vi "GetAllPositions.vi"(8 "error In":errorcluster, 9 "Device Address In":i32, 10 "DeviceKey In":string, 11 "CmdLib In":refnum<k24>) -> (0 "error out":errorcluster, 1 "Device Address Out":i32, 2 "DeviceKey Out":string, 3 "CmdLib Out":refnum<k24>, 4 "Positions":i32[](array[numeric]))   [LabVIEW 2013]
uses:
  C:/GEECS/Developers Version/source/Device Driver/Picomotor8742dotNet/NewFocus/CmdLib.dll
  CmdLib.dll
panel:
  # "Position Motor 1"
  # "Position Motor 2"
  # "Position Motor 3"
  # "Position Motor 4"
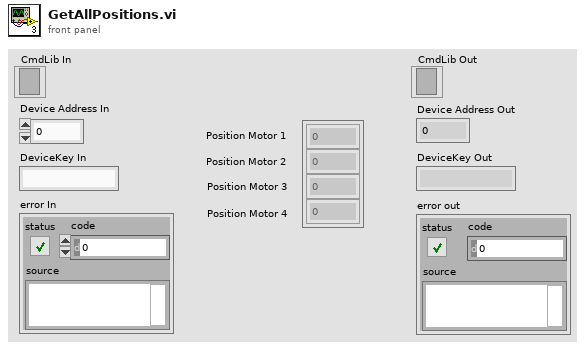
[diagram p1: front panel]
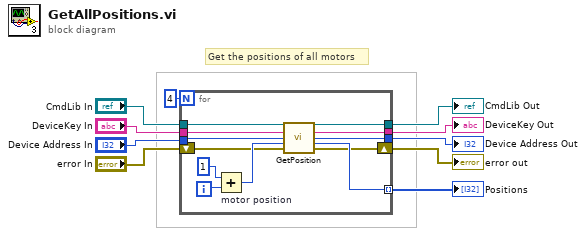
[diagram p0: block diagram]
diagram:
  # "Get the positions of all motors"
  n1 = for {
    N: 4 -> [_]
    tunnel: [w16] -> w9 mode=indexing
    tunnel: "DeviceKey In" -> [w18]
    tunnel: "CmdLib In" -> [w11]
    tunnel: [w17] -> w7
    tunnel: [w14] -> w8
    shift-right: [w15] -> w2
    shift-left: "error In" -> [w19]
    tunnel: "Device Address In" -> [w12]
    tunnel: [w13] -> w6
    i -> [w22]
    n2 = Add "motor position"(x=1 ("y"), y=w22) -> (x+y=w20:i32)
    n3 = call "GetPosition.vi"("CmdLib In"=w11, "DeviceKey In"=w18, "Device Address In"=w12, "Motor"=w20, "error in (no error)"=w19) -> ("CmdLib Out"=w17:refnum<k24>, "DeviceKey Out"=w14:string, "Device Address Out"=w13:i32, "Position"=w16:i32, "error out"=w15:errorcluster)  [unwired: 6 in]
  }
  "Positions" <- w9
  "error out" <- w2
  "DeviceKey Out" <- w8
  "CmdLib Out" <- w7
  "Device Address Out" <- w6
